vi "MakeHTML.vi"(3 "Escape Contents":bool, 4 "HTML Content":string) -> (1 "HTML Element":string)   [LabVIEW 2017, in "ArgosLib.lvlib"]
uses:
  ArgosLib.lvlib
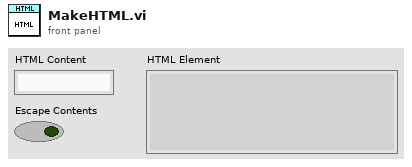
[diagram p1: front panel]
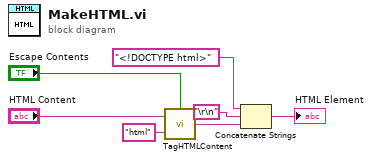
[diagram p0: block diagram]
diagram:
  n1 = call "TagHTMLContent.vi"("Escape Contents"="Escape Contents", "Tag"="html", "Element Contents"="HTML Content") -> ("Tagged Contents"=w3:string)
  n2 = Concatenate Strings("<!DOCTYPE html>" ("string"), "\r\n", w3) -> (→"HTML Element":string)
